vi "WS105x_NI_6501_Relay_Control.vi"(4 "Ring":u16(ring) items=["All Off", "Bank 1", "Bank 2", "Bank 3"], 10 "Relay_ 11":bool, 11 "error in (no error)":errorcluster, 14 "Relay_ 10":bool) -> (0 "RF_SWitch_Ctrl1":bool=TRUE, 1 "RF_SWitch_Ctrl3":bool=TRUE, 2 "RL_3_SW_PIC":bool, 3 "RF_SWitch_Ctrl6":bool=TRUE, 5 "RF_SWitch_Ctrl2":bool=TRUE, 7 "RL_1_SW_PIC":bool, 9 "RL_2_SW_PIC":bool, 12 "RF_SWitch_Ctrl4":bool=TRUE, 13 "RF_SWitch_Ctrl5":bool=TRUE, 15 "error out":errorcluster)   [LabVIEW 2012]
doc: "I. Description:\nThis example demonstrates how to write values to a digital output channel.\n\nII. Instructions for Running:\n1. Select the digital lines on the DAQ device to be written.\n2. Select a value to write.\nNote: The array control is sized for 8 lines, if using a different amount of lines, change the number of elements in the array to equal the number of lines chosen.\n\nIII. Block Diagram Steps:\n1. Create a Digital Output channel. Use one channel for all lines. You can alternatively use one channel for each line, but then use a different polymorphic version of the DAQmx Write VI.\n2. Call the Start VI to start the task.\n3. Write the digital Boolean array data in a loop until the user hits the stop button or an error occurs. This write VI writes a single sample of digital data on demand, so no timeout is necessary.\n4. Call the Clear Task VI to clear the Task.\n5. Use the popup dialog box to display an error or warning if any.\n\nIV. I/O Connections Overview:\nMake sure your signal output terminals match the Lines I/O Control. In this case wire the item to receive the signal to the first eight digital lines on your DAQ Device."
uses:
  <vilib>/DAQmx/create/channels.llb/DAQmx Create Channel (DO-Digital Output).vi
  <vilib>/DAQmx/write.llb/DAQmx Write (Digital Bool 1Line 1Point).vi
panel:
  in  "Lines 11":tag="Dev1/port0/line1" caption="Lines"
  in  "Lines 10":tag="Dev1/port1/line2" caption="Lines"
  in  "Lines 9":tag="Dev1/port1/line4" caption="Lines"
  in  "Lines 8":tag="Dev1/port2/line7" caption="Lines"
  in  "Lines 7":tag="Dev1/port2/line6" caption="Lines"
  in  "Lines 6":tag="Dev1/port2/line5" caption="Lines"
  in  "Lines 5":tag="Dev1/port2/line4" caption="Lines"
  in  "Lines 4":tag="Dev1/port2/line3" caption="Lines"
  in  "Lines 3":tag="Dev1/port2/line2" caption="Lines"
  in  "Lines 2":tag="Dev1/port2/line1" caption="Lines"
  in  "Lines":tag="Dev1/port2/line0"
  # "For instructions, select Help>>Show Context Help"
  # "Channel Parameters"
  # "Pin16"
  # "Pin 14"
  # "Pin 11"
  # "Line 0"
  # "Line 2"
  # "Line 5"
  # "Pin 15"
  # "Pin 13"
  # "Pin 09"
  # "Line 3"
  # "Line 1"
  # "Line 7"
  # "Pin 12"
  # "Pin 6"
  # "Pin 10"
  # "Line 4 Port1"
  # "Line 6"
  # "Line 4"
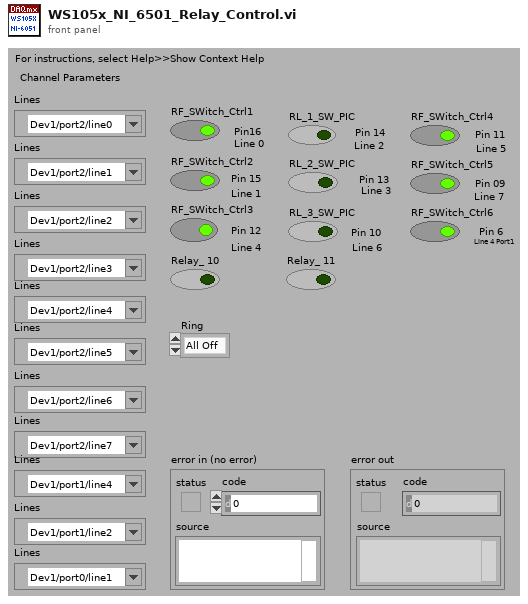
[diagram p1: front panel]
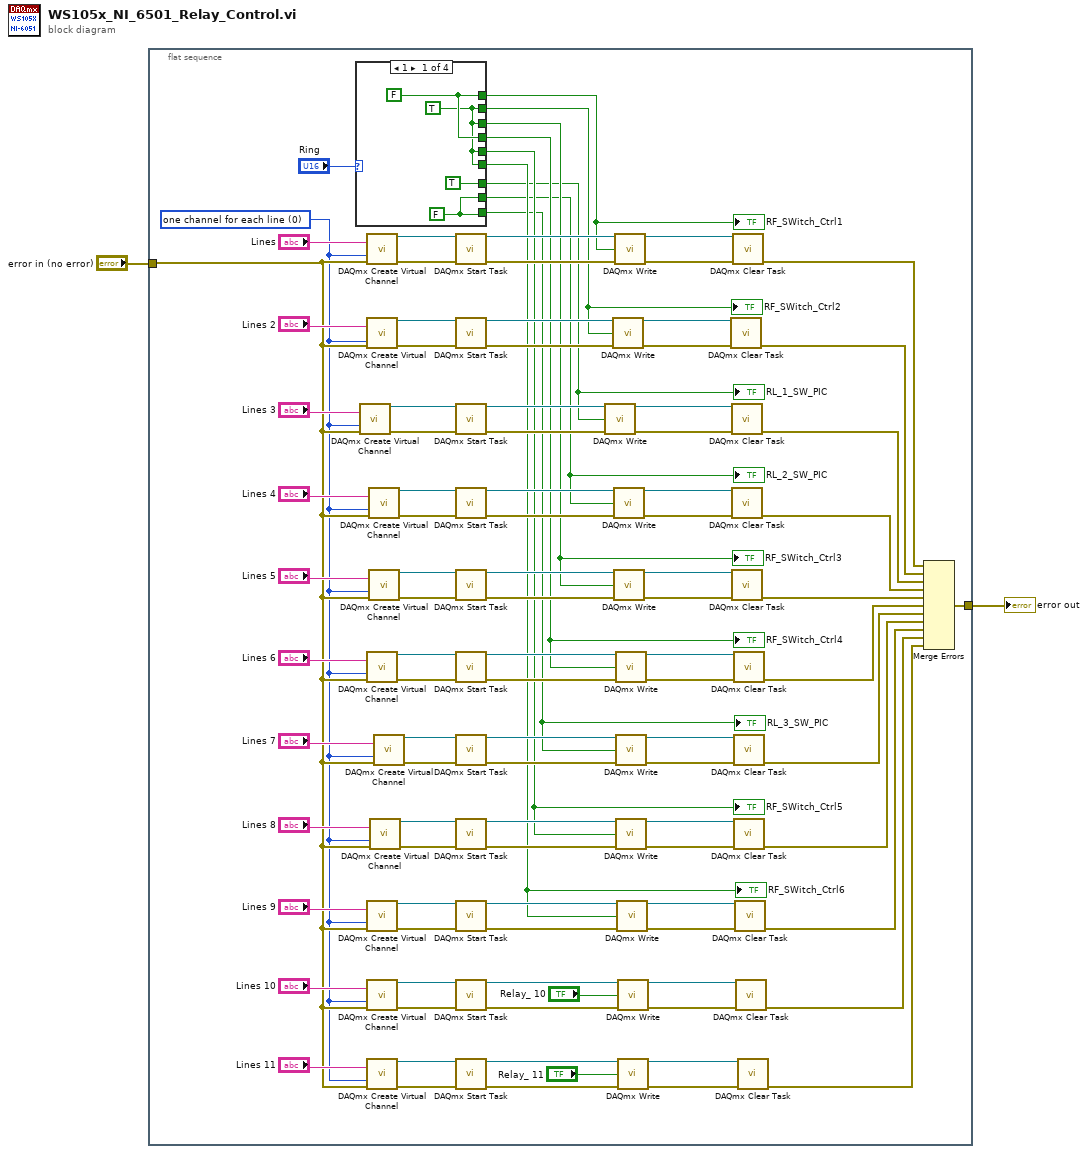
[diagram p0: block diagram]
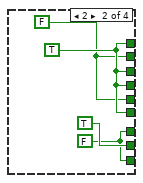
[diagram p2: hidden frame]
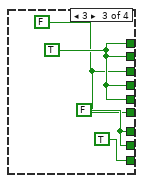
[diagram p3: hidden frame]
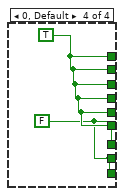
[diagram p4: hidden frame]
diagram:
  n1 = flat-sequence {
    tunnel: "error in (no error)" -> [w16]
    tunnel: [w3] -> w1
    frame #0 {
      w15 = 0 items=["one channel for each line", "one channel for all lines"] ("line grouping")
      n2 = case shown="1" "Ring" {
        tunnel: [w109 w113 w115 w119] -> w34
        tunnel: [w108 w112 w115 w119] -> w33
        tunnel: [w108 w113 w114 w119] -> w32
        tunnel: [w109 w113 w115 w119] -> w31
        tunnel: [w108 w112 w115 w119] -> w30
        tunnel: [w108 w113 w114 w119] -> w29
        tunnel: [TRUE ("RF_SWitch_Ctrl1") w110 w117 w118] -> w28
        tunnel: [w106 TRUE ("RF_SWitch_Ctrl1") w117 w118] -> w27
        tunnel: [w106 w110 TRUE ("RF_SWitch_Ctrl1") w118] -> w26
        frame 1 {
          w106 = FALSE ("RF_SWitch_Ctrl1")
          w108 = TRUE ("RF_SWitch_Ctrl1")
          w109 = FALSE ("RF_SWitch_Ctrl1")
        }
        frame 2 {
          w110 = FALSE ("RF_SWitch_Ctrl1")
          w113 = TRUE ("RF_SWitch_Ctrl1")
          w112 = FALSE ("RF_SWitch_Ctrl1")
        }
        frame 3 {
          w117 = FALSE ("RF_SWitch_Ctrl1")
          w115 = TRUE ("RF_SWitch_Ctrl1")
          w114 = FALSE ("RF_SWitch_Ctrl1")
        }
        frame 0, Default {
          w119 = TRUE ("RF_SWitch_Ctrl1")
          w118 = FALSE ("RF_SWitch_Ctrl1")
        }
      }
      "RF_SWitch_Ctrl1" <- w34
      "RF_SWitch_Ctrl2" <- w33
      "RL_1_SW_PIC" <- w28
      "RF_SWitch_Ctrl3" <- w32
      "RL_2_SW_PIC" <- w27
      "RF_SWitch_Ctrl4" <- w31
      "RF_SWitch_Ctrl5" <- w30
      "RL_3_SW_PIC" <- w26
      "RF_SWitch_Ctrl6" <- w29
      n3 = call-poly <vilib>:"DAQmx Create Virtual Channel.vi"("lines"="Lines 3", "line grouping"=w15, "error in"=w16) -> ("task out"=w87:refnum<k21>, "error out"=w86:errorcluster)  [unwired: 11 in]
      n4 = call-poly <vilib>:"DAQmx Create Virtual Channel.vi"("lines"="Lines", "line grouping"=w15, "error in"=w16) -> ("task out"=w101:refnum<k21>, "error out"=w100:errorcluster)  [unwired: 11 in]
      n5 = call-poly <vilib>:"DAQmx Create Virtual Channel.vi"("lines"="Lines 2", "line grouping"=w15, "error in"=w16) -> ("task out"=w96:refnum<k21>, "error out"=w97:errorcluster)  [unwired: 11 in]
      n6 = call-poly <vilib>:"DAQmx Create Virtual Channel.vi"("lines"="Lines 6", "line grouping"=w15, "error in"=w16) -> ("task out"=w68:refnum<k21>, "error out"=w69:errorcluster)  [unwired: 11 in]
      n7 = call-poly <vilib>:"DAQmx Create Virtual Channel.vi"("lines"="Lines 9", "line grouping"=w15, "error in"=w16) -> ("task out"=w59:refnum<k21>, "error out"=w58:errorcluster)  [unwired: 11 in]
      n8 = call-poly <vilib>:"DAQmx Create Virtual Channel.vi"("lines"="Lines 10", "line grouping"=w15, "error in"=w16) -> ("task out"=w40:refnum<k21>, "error out"=w41:errorcluster)  [unwired: 11 in]
      n9 = call-poly <vilib>:"DAQmx Create Virtual Channel.vi"("lines"="Lines 11", "line grouping"=w15, "error in"=w16) -> ("task out"=w19:refnum<k21>, "error out"=w18:errorcluster)  [unwired: 11 in]
      n10 = call-poly <vilib>:"DAQmx Create Virtual Channel.vi"("lines"="Lines 4", "line grouping"=w15, "error in"=w16) -> ("task out"=w82:refnum<k21>, "error out"=w83:errorcluster)  [unwired: 11 in]
      n11 = call-poly <vilib>:"DAQmx Create Virtual Channel.vi"("lines"="Lines 5", "line grouping"=w15, "error in"=w16) -> ("task out"=w73:refnum<k21>, "error out"=w72:errorcluster)  [unwired: 11 in]
      n12 = call-poly <vilib>:"DAQmx Create Virtual Channel.vi"("lines"="Lines 8", "line grouping"=w15, "error in"=w16) -> ("task out"=w54:refnum<k21>, "error out"=w55:errorcluster)  [unwired: 11 in]
      n13 = call-poly <vilib>:"DAQmx Create Virtual Channel.vi"("lines"="Lines 7", "line grouping"=w15, "error in"=w16) -> ("task out"=w45:refnum<k21>, "error out"=w44:errorcluster)  [unwired: 11 in]
      n14 = call <vilib>:"DAQmx Start Task.vi"("task/channels in"=w101, "error in"=w100) -> ("task out"=w103:refnum<k21>, "error out"=w105:errorcluster)  [unwired: 12 in]
      n15 = call <vilib>:"DAQmx Start Task.vi"("task/channels in"=w96, "error in"=w97) -> ("task out"=w94:refnum<k21>, "error out"=w92:errorcluster)  [unwired: 12 in]
      n16 = call <vilib>:"DAQmx Start Task.vi"("task/channels in"=w87, "error in"=w86) -> ("task out"=w89:refnum<k21>, "error out"=w91:errorcluster)  [unwired: 12 in]
      n17 = call <vilib>:"DAQmx Start Task.vi"("task/channels in"=w82, "error in"=w83) -> ("task out"=w80:refnum<k21>, "error out"=w78:errorcluster)  [unwired: 12 in]
      n18 = call <vilib>:"DAQmx Start Task.vi"("task/channels in"=w73, "error in"=w72) -> ("task out"=w75:refnum<k21>, "error out"=w77:errorcluster)  [unwired: 12 in]
      n19 = call <vilib>:"DAQmx Start Task.vi"("task/channels in"=w68, "error in"=w69) -> ("task out"=w66:refnum<k21>, "error out"=w64:errorcluster)  [unwired: 12 in]
      n20 = call <vilib>:"DAQmx Start Task.vi"("task/channels in"=w45, "error in"=w44) -> ("task out"=w47:refnum<k21>, "error out"=w49:errorcluster)  [unwired: 12 in]
      n21 = call <vilib>:"DAQmx Start Task.vi"("task/channels in"=w54, "error in"=w55) -> ("task out"=w52:refnum<k21>, "error out"=w50:errorcluster)  [unwired: 12 in]
      n22 = call <vilib>:"DAQmx Start Task.vi"("task/channels in"=w59, "error in"=w58) -> ("task out"=w61:refnum<k21>, "error out"=w63:errorcluster)  [unwired: 12 in]
      n23 = call <vilib>:"DAQmx Start Task.vi"("task/channels in"=w40, "error in"=w41) -> ("task out"=w38:refnum<k21>, "error out"=w36:errorcluster)  [unwired: 12 in]
      n24 = call <vilib>:"DAQmx Start Task.vi"("task/channels in"=w19, "error in"=w18) -> ("task out"=w21:refnum<k21>, "error out"=w23:errorcluster)  [unwired: 12 in]
      n25 = call-poly <vilib>:"DAQmx Write.vi"("task/channels in"=w89, "data"=w28, "error in"=w91) -> ("task out"=w88:refnum<k21>, "error out"=w90:errorcluster)  [unwired: 10 in, 1 out]
      n26 = call-poly <vilib>:"DAQmx Write.vi"("task/channels in"=w94, "data"=w33, "error in"=w92) -> ("task out"=w95:refnum<k21>, "error out"=w93:errorcluster)  [unwired: 10 in, 1 out]
      n27 = call-poly <vilib>:"DAQmx Write.vi"("task/channels in"=w80, "data"=w27, "error in"=w78) -> ("task out"=w81:refnum<k21>, "error out"=w79:errorcluster)  [unwired: 10 in, 1 out]
      n28 = call-poly <vilib>:"DAQmx Write.vi"("task/channels in"=w75, "data"=w32, "error in"=w77) -> ("task out"=w74:refnum<k21>, "error out"=w76:errorcluster)  [unwired: 10 in, 1 out]
      n29 = call-poly <vilib>:"DAQmx Write.vi"("task/channels in"=w103, "data"=w34, "error in"=w105) -> ("task out"=w102:refnum<k21>, "error out"=w104:errorcluster)  [unwired: 10 in, 1 out]
      n30 = call-poly <vilib>:"DAQmx Write.vi"("task/channels in"=w66, "data"=w31, "error in"=w64) -> ("task out"=w67:refnum<k21>, "error out"=w65:errorcluster)  [unwired: 10 in, 1 out]
      n31 = call-poly <vilib>:"DAQmx Write.vi"("task/channels in"=w47, "data"=w26, "error in"=w49) -> ("task out"=w46:refnum<k21>, "error out"=w48:errorcluster)  [unwired: 10 in, 1 out]
      n32 = call-poly <vilib>:"DAQmx Write.vi"("task/channels in"=w52, "data"=w30, "error in"=w50) -> ("task out"=w53:refnum<k21>, "error out"=w51:errorcluster)  [unwired: 10 in, 1 out]
      n33 = call-poly <vilib>:"DAQmx Write.vi"("task/channels in"=w61, "data"=w29, "error in"=w63) -> ("task out"=w60:refnum<k21>, "error out"=w62:errorcluster)  [unwired: 10 in, 1 out]
      n34 = call-poly <vilib>:"DAQmx Write.vi"("task/channels in"=w38, "data"="Relay_ 10", "error in"=w36) -> ("task out"=w39:refnum<k21>, "error out"=w37:errorcluster)  [unwired: 10 in, 1 out]
      n35 = call-poly <vilib>:"DAQmx Write.vi"("task/channels in"=w21, "data"="Relay_ 11", "error in"=w23) -> ("task out"=w20:refnum<k21>, "error out"=w22:errorcluster)  [unwired: 10 in, 1 out]
      n36 = call <vilib>:"DAQmx Clear Task.vi"("task in"=w95, "error in"=w93) -> ("error out"=w13:errorcluster)  [unwired: 13 in]
      n37 = call <vilib>:"DAQmx Clear Task.vi"("task in"=w88, "error in"=w90) -> ("error out"=w12:errorcluster)  [unwired: 13 in]
      n38 = call <vilib>:"DAQmx Clear Task.vi"("task in"=w81, "error in"=w79) -> ("error out"=w11:errorcluster)  [unwired: 13 in]
      n39 = call <vilib>:"DAQmx Clear Task.vi"("task in"=w74, "error in"=w76) -> ("error out"=w10:errorcluster)  [unwired: 13 in]
      n40 = call <vilib>:"DAQmx Clear Task.vi"("task in"=w102, "error in"=w104) -> ("error out"=w14:errorcluster)  [unwired: 13 in]
      n41 = call <vilib>:"DAQmx Clear Task.vi"("task in"=w67, "error in"=w65) -> ("error out"=w9:errorcluster)  [unwired: 13 in]
      n42 = call <vilib>:"DAQmx Clear Task.vi"("task in"=w46, "error in"=w48) -> ("error out"=w8:errorcluster)  [unwired: 13 in]
      n43 = call <vilib>:"DAQmx Clear Task.vi"("task in"=w53, "error in"=w51) -> ("error out"=w7:errorcluster)  [unwired: 13 in]
      n44 = call <vilib>:"DAQmx Clear Task.vi"("task in"=w60, "error in"=w62) -> ("error out"=w6:errorcluster)  [unwired: 13 in]
      n45 = call <vilib>:"DAQmx Clear Task.vi"("task in"=w39, "error in"=w37) -> ("error out"=w5:errorcluster)  [unwired: 13 in]
      n46 = call <vilib>:"DAQmx Clear Task.vi"("task in"=w20, "error in"=w22) -> ("error out"=w4:errorcluster)  [unwired: 13 in]
      n47 = Merge Errors(w14, w13, w12, w11, w10, w9, w8, w7, w6, w5, w4) -> (w3:errorcluster)
    }
  }
  "error out" <- w1
